vi "EventLoop.MATLAB.vi"(0 "Path":path) -> ()   [LabVIEW 2014]
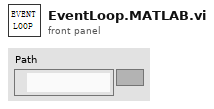
[diagram p1: front panel]
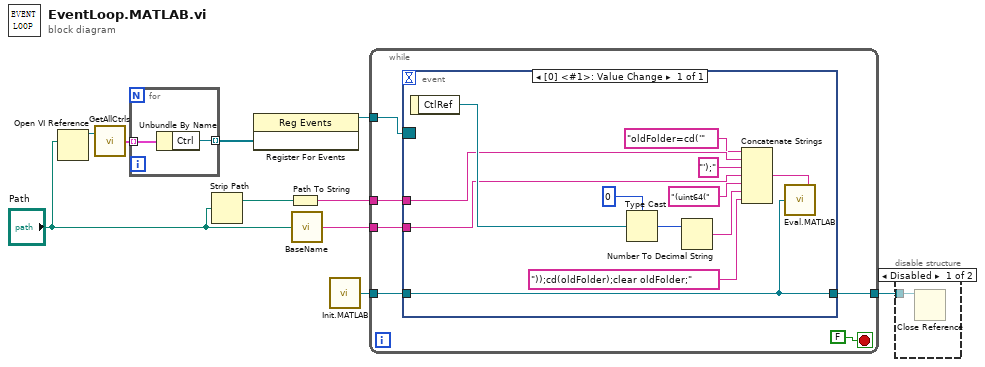
[diagram p0: block diagram]
diagram:
  n1 = Open VI Reference(vi path="Path") -> (vi reference=w4:refnum<vi>)  [unwired: 5 in, 1 out]
  n2 = call "GetAllCtrls.vi"("VI"=w4) -> ("Ctrls"=w5:cluster{"Name":string, "Ctrl":refnum<vi>}[])  [unwired: 1 in]
  n3 = for {
    tunnel: w5 -> [w12] mode=indexing
    tunnel: [w11] -> w9 mode=indexing
    n4 = Unbundle By Name(w12) -> ("Ctrl"=w11:refnum<vi>)
  }
  n5 = Strip Path(path="Path") -> (stripped path=w2:path)  [unwired: 1 out]
  n6 = register-events(w9) -> (reference out=w10:refnum<event-registration>)  [unwired: 2 in, 1 out]
  n7 = Path To String(path=w2) -> (string=w1:string)
  n8 = call "BaseName.vi"("Path"="Path") -> ("Name"=w7:string)
  n9 = call "Init.MATLAB.vi"() -> ("reference"=w6:refnum<k24>)
  n10 = while {
    tunnel: w6 -> [w17]
    tunnel: w10 -> [w16]
    tunnel: [w15] -> w8
    tunnel: w7 -> [w14]
    tunnel: w1 -> [w13]
    stop <- FALSE stop-if-true
    n11 = event shown="[0] <#1>: Value Change" {
      selector: w16 -> [_]
      dyn-events: _ -> [_]
      timeout: _ -> [_]
      tunnel: w17 -> [w23]
      tunnel: [w23] -> w15
      tunnel: w14 -> [w24]
      tunnel: w13 -> [w20]
      event Value Change {
        n12 = event-data() -> ("CtlRef"=w29:refnum<vi>)  [unwired: 1 in]
        n13 = Type Cast(type=u32 0, x=w29) -> (*(type *) &x=w28:u32)
        n14 = Number To Decimal String(number=w28) -> (decimal integer string=w27:string)  [unwired: 1 in]
        n15 = Concatenate Strings("oldFolder=cd('" ("string"), w20, "');" ("string"), w24, "(uint64(" ("string"), w27, "));cd(oldFolder);clear oldFolder;" ("string")) -> (w22:string)
        n16 = call "Eval.MATLAB.vi"("input"=w22, "reference"=w23) -> ()
      }
    }
  }
  n17 = disable-structure shown="Disabled" {
    disable-tunnel: w8 -> [w31 _]
    frame Disabled {
      n18 = Close Reference(reference=w31) -> ()  [unwired: 1 in, 1 out]
    }
    frame Enabled {
    }
  }
